vi "Save_Measurement_data.vi"(6 "Mergedata_struct":refnum<k24>[](array[refnum]), 7 "ILSTS":refnum<k24>, 8 "错误输入（无错误）":errorcluster, 9 "Data_struct":refnum<k24>[](array[refnum])) -> (0 "错误输出":errorcluster)   [LabVIEW 2017]
doc: "Save Measurement data"
uses:
  D:/test/ILSTS/LV_IL/LV_IL_Sample_x64/DLL/STSProcess.dll
  DLL/STSProcess.dll
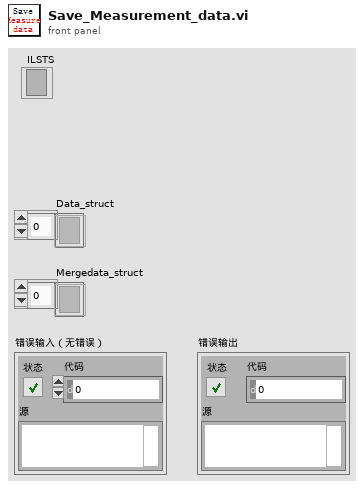
[diagram p1: front panel]
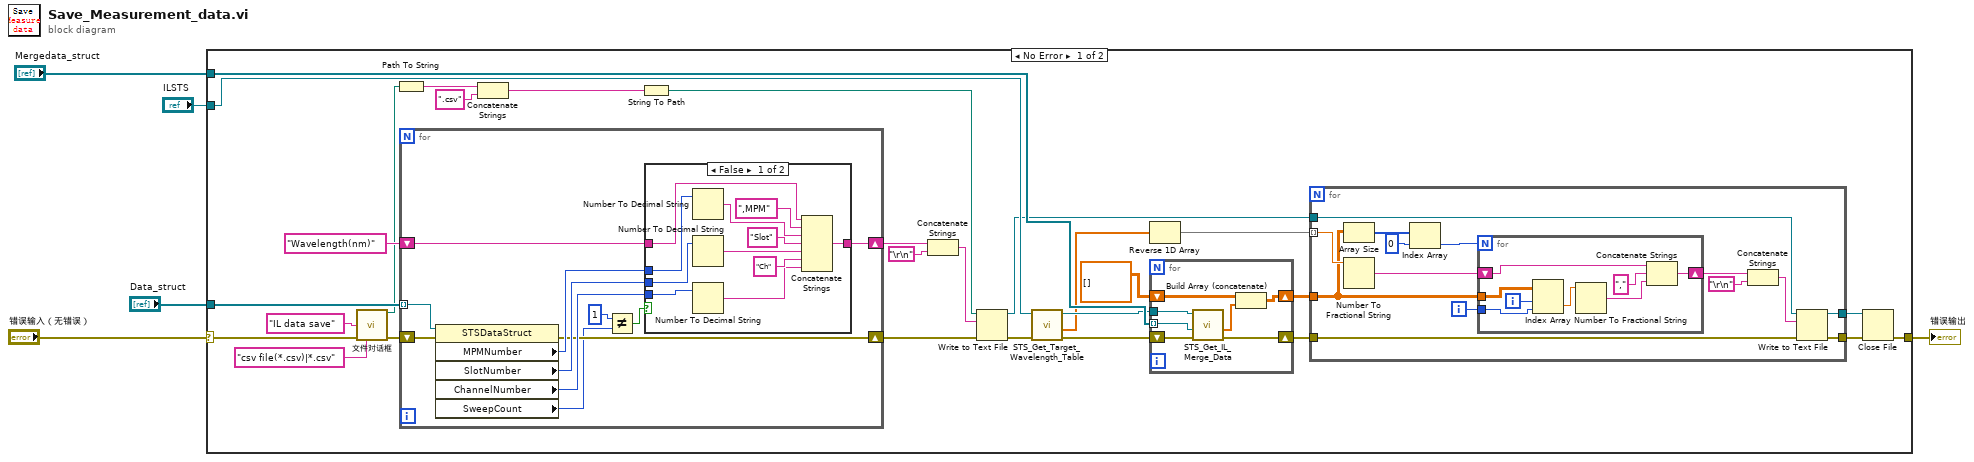
[diagram p0: block diagram]
diagram:
  n1 = case shown="No Error" "错误输入（无错误）" {
    selector: "错误输入（无错误）" -> [w30 w87]
    tunnel: "Data_struct" -> [w22 _]
    tunnel: [w14 w87] -> w4
    tunnel: "Mergedata_struct" -> [w34 _]
    tunnel: "ILSTS" -> [w33 _]
    frame No Error {
      n2 = call "文件对话框"("default name"="IL data save" ("字符串"), "error in"=w30, "pattern (all files)"="csv file(*.csv)|*.csv") -> ("selected path"=w20:path, "error out"=w23:errorcluster)  [unwired: 9 in, 2 out]
      n3 = Path To String(path=w20) -> (string=w19:string)
      n4 = for {
        tunnel: w22 -> [w74] mode=indexing
        shift-right: [w68] -> w28
        shift-left: "Wavelength(nm)" -> [w69]
        shift-right: [w67] -> w27
        shift-left: w23 -> [w73]
        n5 = property on="属性节点" class="STSDataStruct"(reference=w74, error in=w73) -> (error out=w67:errorcluster, "MPMNumber"=w70:i32, "SlotNumber"=w71:i32, "ChannelNumber"=w72:i32, "SweepCount"=w66:i32)  [unwired: 1 out]
        n6 = Not Equal?(x=1, y=w66) -> (x != y?=w64:bool)
        n7 = case shown="False" w64 {
          tunnel: w72 -> [w85 _]
          tunnel: w71 -> [w84 _]
          tunnel: w70 -> [w83 _]
          tunnel: w69 -> [w82 w86]
          tunnel: [w75 w86] -> w68
          frame False {
            n8 = Number To Decimal String(number=w83) -> (decimal integer string=w80:string)  [unwired: 1 in]
            n9 = Number To Decimal String(number=w84) -> (decimal integer string=w78:string)  [unwired: 1 in]
            n10 = Number To Decimal String(number=w85) -> (decimal integer string=w76:string)  [unwired: 1 in]
            n11 = Concatenate Strings(w82, ",MPM" ("字符串"), w80, "Slot" ("字符串"), w78, "Ch" ("字符串"), w76) -> (w75:string)
          }
          frame True {
          }
        }
      }
      n12 = Concatenate Strings(w19, ".csv" ("名称或相对路径")) -> (w17:string)
      n13 = String To Path(string=w17) -> (path=w16:path)
      n14 = Concatenate Strings(w28, "\r\n") -> (w29:string)
      n15 = Write to Text File(file (use dialog)=w16, text=w29, error in=w27) -> (refnum out=w24:refnum<file>, error out=w21:errorcluster)  [unwired: 1 in, 1 out]
      n16 = call "STS_Get_Target_Wavelength_Table.vi"("错误输入（无错误）"=w21, ".NET引用句柄输入"=w33) -> ("error out"=w12:errorcluster, "wavelengths"=w7:dbl[], "引用输出"=w11:refnum<k24>)  [unwired: 7 in]
      n17 = Reverse 1D Array(array=w7) -> (reversed array=w6:dbl[])
      n18 = for {
        tunnel: w11 -> [w62]
        tunnel: w34 -> [w61] mode=indexing
        shift-right: [w60] -> w8
        shift-left: w12 -> [w63]
        shift-right: [w57] -> w9
        shift-left: sgl[][] [] -> [w58]
        n19 = call "STS_Get_IL_Merge_Data.vi"("错误输入（无错误）"=w63, "setting"=w61, ".NET引用句柄输入"=w62) -> ("error out"=w60:errorcluster, "ilData"=w59:sgl[])  [unwired: 6 in, 1 out]
        n20 = Build Array (concatenate)(w58, w59) -> (w57:sgl[][])
      }
      n21 = for {
        tunnel: w6 -> [w48] mode=indexing
        tunnel: w9 -> [w45]
        tunnel: w8 -> [w44]
        tunnel: [w43] -> w15
        tunnel: w24 -> [w36]
        tunnel: [w35] -> w13
        i -> [w47]
        n22 = Array Size(array=w45) -> (size(s)=w39:i32[])
        n23 = Number To Fractional String(number=w48) -> (F-format string=w46:string)  [unwired: 3 in]
        n24 = Index Array(array=w39, index=0 ("索引")) -> (element=w37:i32)
        n25 = for {
          N: w37 -> [_]
          tunnel: w45 -> [w56]
          tunnel: w47 -> [w55]
          shift-right: [w51] -> w42
          shift-left: w46 -> [w52]
          i -> [w54]
          n26 = Index Array(array=w56, index (row)=w54, index (col)=w55) -> (element=w53:sgl)
          n27 = Number To Fractional String(number=w53) -> (F-format string=w49:string)  [unwired: 3 in]
          n28 = Concatenate Strings(w52, "," ("字符串"), w49) -> (w51:string)
        }
        n29 = Concatenate Strings(w42, "\r\n") -> (w40:string)
        n30 = Write to Text File(file (use dialog)=w36, text=w40, error in=w44) -> (refnum out=w35:refnum<file>, error out=w43:errorcluster)  [unwired: 1 in, 1 out]
      }
      n31 = Close File(refnum=w13, error in=w15) -> (error out=w14:errorcluster)  [unwired: 1 out]
    }
    frame Error {
    }
  }
  "错误输出" <- w4
